vi "Write Object Coordinate.vi"(10 "Object Coordinate":cluster{"Horizontal":i32, "Vertical":i32}, 11 "Mouse in":refnum<class "Mouse.lvclass">) -> (3 "Mouse out":refnum<class "Mouse.lvclass">)   [LabVIEW 2021, in "Mouse.lvclass"]
doc: "MIT Licence\nCopyright (c) 2024 David Grollier"
uses:
  Mouse.lvclass
  Mouse.lvclass/Mouse.ctl
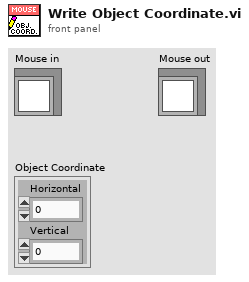
[diagram p1: front panel]
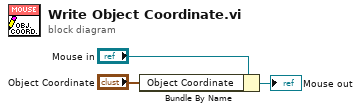
[diagram p0: block diagram]
diagram:
  n1 = Bundle By Name(cluster="Mouse in", "Object Coordinate"="Object Coordinate") -> (→"Mouse out":refnum<class "Mouse.lvclass">)
